vi "Loop_Start.vi"(2 "Command":cluster{string, string[], dbl[], dbl}, 3 "Loop Count In":cluster{string, "Position":i32}[](array[cluster])) -> (0 "Ended Loop":cluster{string, "Position":i32}[](array[cluster]), 1 "Loop Count Out":cluster{string, "Position":i32}[](array[cluster]))   [LabVIEW 2011]
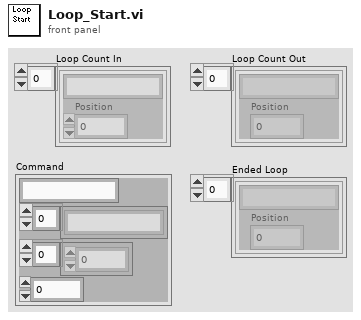
[diagram p1: front panel]
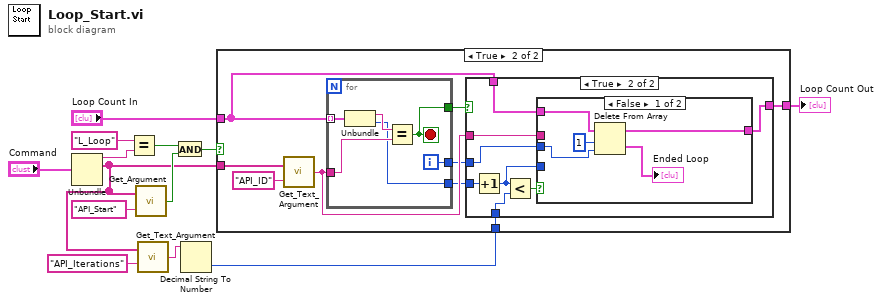
[diagram p0: block diagram]
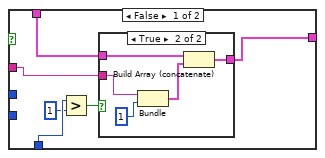
[diagram p3: hidden frame]
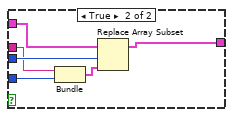
[diagram p5: hidden frame]
diagram:
  n1 = Unbundle("Command") -> (w12:string, w4:string[])  [unwired: 2 out]
  n2 = Equal?(x="L_Loop", y=w12) -> (x = y?=w9:bool)
  n3 = call "Get_Argument.vi"("Argument"="API_Start", "Argument List"=w4) -> ("Enabled"=w8:bool)
  n4 = call "Get_Text_Argument.vi"("Argument"="API_Iterations", "Argument List"=w4) -> ("Text"=w2:string)
  n5 = And(x=w9, y=w8) -> (x .and. y?=w7:bool)
  n6 = Decimal String To Number(string=w2) -> (number=w1:i32)  [unwired: 2 in, 1 out]
  n7 = case shown="True" w7 {
    tunnel: "Loop Count In" -> [w14 w20]
    tunnel: w4 -> [_ w23]
    tunnel: [w14 w18] -> w5
    tunnel: w1 -> [_ w17]
    frame False {
    }
    frame True {
      n8 = call "Get_Text_Argument.vi"("Argument"="API_ID", "Argument List"=w23) -> ("Text"=w19:string)
      n9 = for {
        tunnel: w20 -> [w60] mode=indexing
        tunnel: w19 -> [w57]
        tunnel: [w58] -> w21
        tunnel: [w56] -> w16
        tunnel: [w55] -> w15
        i -> [w55]
        stop <- w58 stop-if-true
        n10 = Unbundle(w60) -> (w59:string, "Position"=w56:i32)
        n11 = Equal?(x=w59, y=w57) -> (x = y?=w58:bool)
      }
      n12 = case shown="True" w21 {
        tunnel: w20 -> [w29 w42]
        tunnel: w19 -> [w28 w40]
        tunnel: [w27 w39] -> w18
        tunnel: w17 -> [w25 w43]
        tunnel: w16 -> [_ w37]
        tunnel: w15 -> [_ w41]
        frame False {
          n13 = Greater?(x=w25, y=1) -> (0:w26:bool)
          n14 = case shown="True" w26 {
            tunnel: w29 -> [w30 w35]
            tunnel: w28 -> [_ w34]
            tunnel: [w30 w31] -> w27
            frame False {
            }
            frame True {
              n15 = Bundle("Text"=w34, "Position"=1) -> (w32:cluster{"Text":string, "Position":i32})  [unwired: 1 in]
              n16 = Build Array (concatenate)(w35, w32) -> (w31:cluster{"Text":string, "Position":i32}[])
            }
          }
        }
        frame True {
          n17 = Increment(x=w37) -> (x+1=w36:i32)
          n18 = Less?(x=w36, y=w43) -> (x < y?=w38:bool)
          n19 = case shown="False" w38 {
            tunnel: w42 -> [w48 w54]
            tunnel: w41 -> [w45 w53]
            tunnel: w40 -> [_ w52]
            tunnel: [w47 w50] -> w39
            tunnel: w36 -> [_ w49]
            frame False {
              n20 = Delete From Array(array=w48, length=1, index=w45) -> (deleted portion=→"Ended Loop":cluster{string, "Position":i32}[], array with subset deleted=w47:cluster{string, "Position":i32}[])
            }
            frame True {
              n21 = Bundle("Text"=w52, w49) -> (w51:cluster{"Text":string, i32})  [unwired: 1 in]
              n22 = Replace Array Subset(array=w54, new element=w51, index=w53) -> (w50:cluster{string, "Position":i32}[])
            }
          }
        }
      }
    }
  }
  "Loop Count Out" <- w5
